vi "SetExitFlag.vi"(8 "error in (no error)":errorcluster, 11 "GUI_Handler_Main in":refnum<class "GUI_Handler_Main.lvclass">) -> (0 "error out":errorcluster, 3 "GUI_Handler_Main out":refnum<class "GUI_Handler_Main.lvclass">)   [LabVIEW 2019, in "GUI_Handler_Main.lvclass"]
uses:
  GUI_Handler_Main.lvclass
  GUI_Handler_Main.lvclass/GUI_Handler_Main.ctl
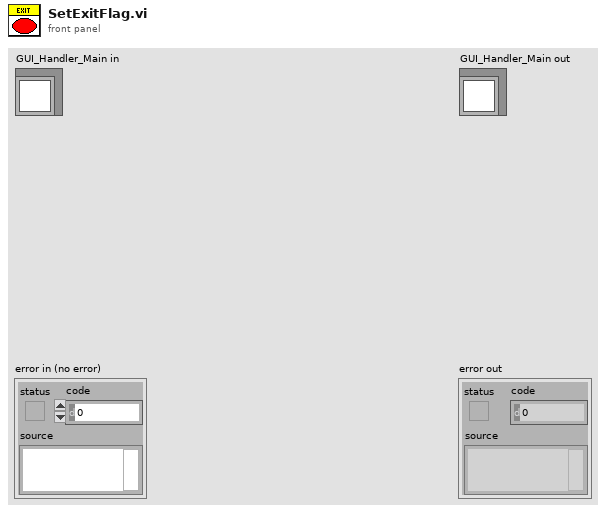
[diagram p1: front panel]
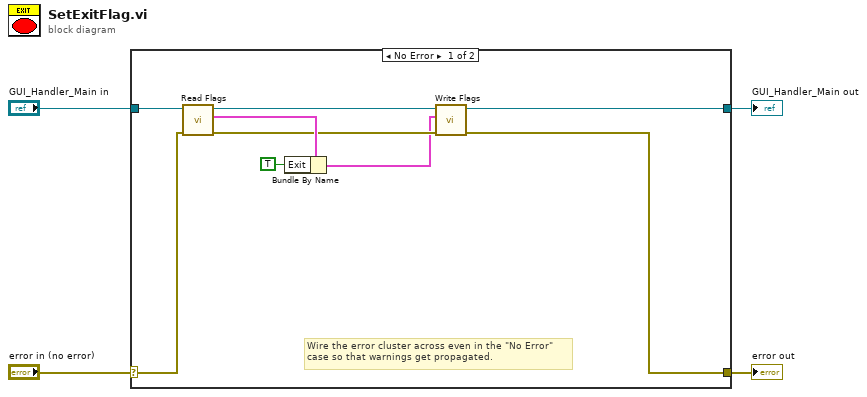
[diagram p0: block diagram]
diagram:
  n1 = case shown="No Error" "error in (no error)" {
    selector: "error in (no error)" -> [w5 w15]
    tunnel: [w6 w15] -> w3
    tunnel: [w9 w14] -> w1
    tunnel: "GUI_Handler_Main in" -> [w13 w14]
    frame No Error {
      # "Wire the error cluster across even in the \"No Error\"\ncase so that warnings get propagated."
      n2 = call "Read Flags.vi"("error in (no error)"=w5, "GUI_Handler_Main in"=w13) -> ("error out"=w8:errorcluster, "Flags"=w12:cluster{"Exit":bool}, "GUI_Handler_Main out"=w10:refnum<class "GUI_Handler_Main.lvclass">)  [unwired: 7 in]
      n3 = Bundle By Name(cluster=w12, "Exit"=TRUE) -> (w7:cluster{"Exit":bool})
      n4 = call "Write Flags.vi"("error in (no error)"=w8, "Flags"=w7, "GUI_Handler_Main in"=w10) -> ("error out"=w6:errorcluster, "GUI_Handler_Main out"=w9:refnum<class "GUI_Handler_Main.lvclass">)  [unwired: 7 in]
    }
    frame Error {
    }
  }
  "error out" <- w3
  "GUI_Handler_Main out" <- w1
